vi "Core.vi"(8 "error in (no error)":errorcluster, 10 "Actor in":refnum<class "Actor.lvclass">, 11 "Timed Msg in":refnum<class "Ping Msg.lvclass">) -> (0 "error out":errorcluster, 1 "Data":refnum<class "Data.lvclass">, 2 "Actor out":refnum<class "Actor.lvclass">, 3 "Timed Msg out":refnum<class "Ping Msg.lvclass">)   [LabVIEW 2020, in "Publisher.lvlib" / "Ping Msg.lvclass"]
doc: "Core of the Reponse Msg. Put the active code here.\n\nThis implementation returns a TRUE wrapped in a Boolean class."
uses:
  Ping Msg.lvclass
  PPL/HDH.Data.Generic.lvlibp/Data.lvclass
  PPL/HDH.Actor Framework.Core.Actor.lvlibp/1abvi3w/vi.lib/ActorFramework/Actor/Actor.lvclass
  PPL/HDH.Data.Generic.lvlibp/Generic Data/Boolean/Boolean.lvclass
  C:/Current projects/WS/PPL/HDH.Data.Generic.lvlibp/Data.lvclass
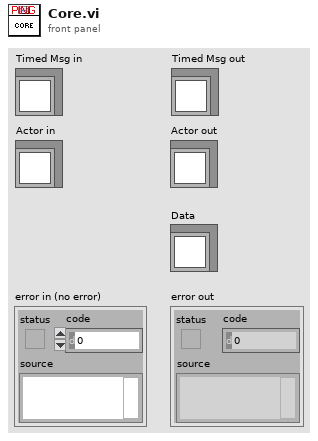
[diagram p1: front panel]
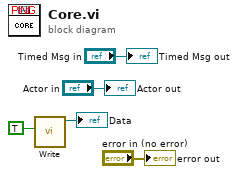
[diagram p0: block diagram]
diagram:
  n1 = call "Write.vi"("Boolean"=TRUE) -> ("Boolean out"=→"Data":refnum<class "Boolean.lvclass">)  [unwired: 10 in]
  "error out" <- "error in (no error)"
  "Actor out" <- "Actor in"
  "Timed Msg out" <- "Timed Msg in"
